vi "GetTreeSetup.vi"(1 "All Folders":path[](array[path])) -> (0 "Format":T1(array[cluster]))   [LabVIEW 2014]
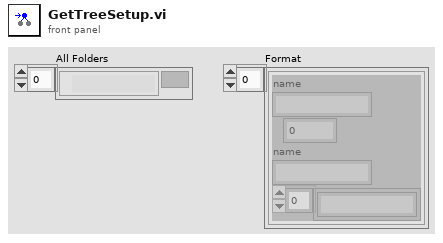
[diagram p1: front panel]
types:
  T1 = cluster{"name":string, i32, "name":string, string[]}[]
  T2 = cluster{"name":string, i32, "name":string, string[]}
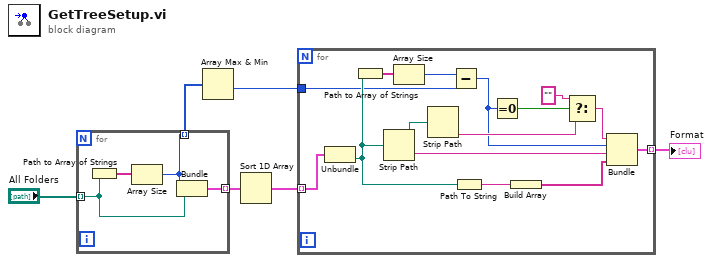
[diagram p0: block diagram]
diagram:
  n1 = for {
    tunnel: "All Folders" -> [w8] mode=indexing
    tunnel: [w10] -> w3 mode=indexing
    tunnel: [w7] -> w2 mode=indexing
    n2 = Path to Array of Strings(0:w8) -> (2:w9:string[])  [unwired: 1 out]
    n3 = Array Size(array=w9) -> (size(s)=w7:i32)
    n4 = Bundle(w7, "Folder Path"=w8) -> (w10:cluster{i32, "Folder Path":path})  [unwired: 1 in]
  }
  n5 = Array Max & Min(array=w2) -> (min value=w1:i32)  [unwired: 3 out]
  n6 = Sort 1D Array(array=w3) -> (sorted array=w4:cluster{i32, "Folder Path":path}[])
  n7 = for {
    tunnel: w4 -> [w25] mode=indexing
    tunnel: [w14] -> w6 mode=indexing
    tunnel: w1 -> [w11]
    n8 = Unbundle(w25) -> ("Folder Path"=w18:path)  [unwired: 1 out]
    n9 = Path to Array of Strings(0:w18) -> (2:w20:string[])  [unwired: 1 out]
    n10 = Strip Path(path=w18) -> (stripped path=w22:path, name=w16:string)
    n11 = Array Size(array=w20) -> (size(s)=w21:i32)
    n12 = Strip Path(path=w22) -> (name=w23:string)  [unwired: 1 out]
    n13 = Subtract(x=w21, y=w11) -> (x-y=w13:i32)
    n14 = Path To String(path=w18) -> (string=w19:string)
    n15 = Equal To 0?(x=w13) -> (x = 0?=w12:bool)
    n16 = Build Array(w19) -> (w15:string[])
    n17 = Select(t="", s=w12, f=w23) -> (s? t:f=w17:string)
    n18 = Bundle("name"=w17, w13, "name"=w16, w15) -> (w14:T2)  [unwired: 1 in]
  }
  "Format" <- w6
